vi "Auton - Boiler Shoot.vi"(10 "Alliance":T2, 11 "Auton States":T1=enum."Reset Encoders") -> ()   [LabVIEW 2016]
uses:
  Auton - Boiler Shoot States.ctl
  <vilib>/Rock Robotics/WPI/DriverStation/WPI_DriverStationAllianceInfo.ctl
  Robot Values.vi
panel:
  out "Auton State Current":T1=enum."Reset Encoders"
  in  "High Speed Output Range":cluster{"output high":dbl, "output low":dbl}={"output high"=0.9, "output low"=-0.9}
  in  "Cross Baseline SP":dbl=50.0
  in  "Turn to Zero SP (...)":dbl format="%#_13g"
  out "Original Time":timestamp
  in  "Back away  SP":dbl
  in  "Red - Turn Toward Angle SP":dbl=128.0
  in  "Approach Boiler SP":dbl=22.0
  in  "Blue - Turn Toward Angle SP":dbl=232.0
  in  "Initial Drive Forward SP":dbl=34.0
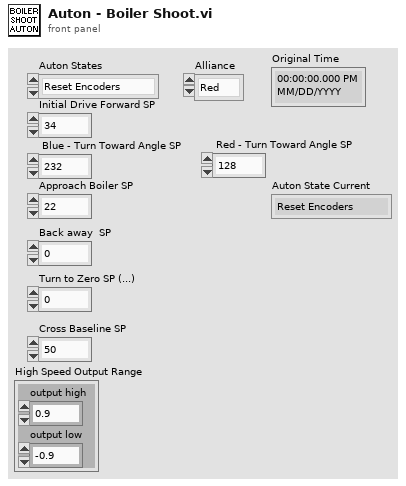
[diagram p1: front panel]
types:
  T1 = typedef "Auton - Boiler Shoot States.ctl" = enum16{"Stop", "Reset Encoders", "Drive Forward", "Turn toward boiler", "Reset Encoders Again", "Drive to boiler", "Shoot", "Back from Boiler", "Turn to Zero", "Reset Encoders Again Again", "Cross Baseline"}
  T2 = typedef "WPI_DriverStationAllianceInfo.ctl" = enum16{"Red", "Blue", "Invalid"}
  T3 = typedef "Robot Values.ctl" = cluster{"Robot Drive":cluster{"Left Motor Power":dbl, "Right Motor Power":dbl, "Left Encoder Value":dbl, "Right Encoder Value":dbl, "High Gear?":bool, "PTO?":bool}, "Sensors":cluster{"Gyro Angle":u16, "Recalibrate Gyro":bool, "Reset Gyro":bool, "Ultrasonic":dbl}, "Shooter":cluster{"Prep Wheels":bool, "Shoot":bool, "Left Shooter Wheel Speed":dbl, "Wheels Moving":bool, "Shooter Prepped":bool, "Shooter RPS SP":dbl, "Shooting?":bool, "Left Shooter Wheel Power":dbl, "Right Shooter Wheel Power":dbl, "Acquisition Conveyor Power":dbl, "Hopper Beater Bar Power":dbl, "Filtered Left Shooter Speed":dbl, "Acquisition Motor Power":dbl, "Joystick Add":dbl, "D-Pad Add":dbl, "Shooter Use PID?":bool}, "Robot States":cluster{"Drive mode":string, "Alliance":T2, "Position":T4}, "Gear":cluster{"Ejection Active":bool}}
  T4 = typedef "WPI_DriverStationPositionInfo.ctl" = enum16{"1", "2", "3"}
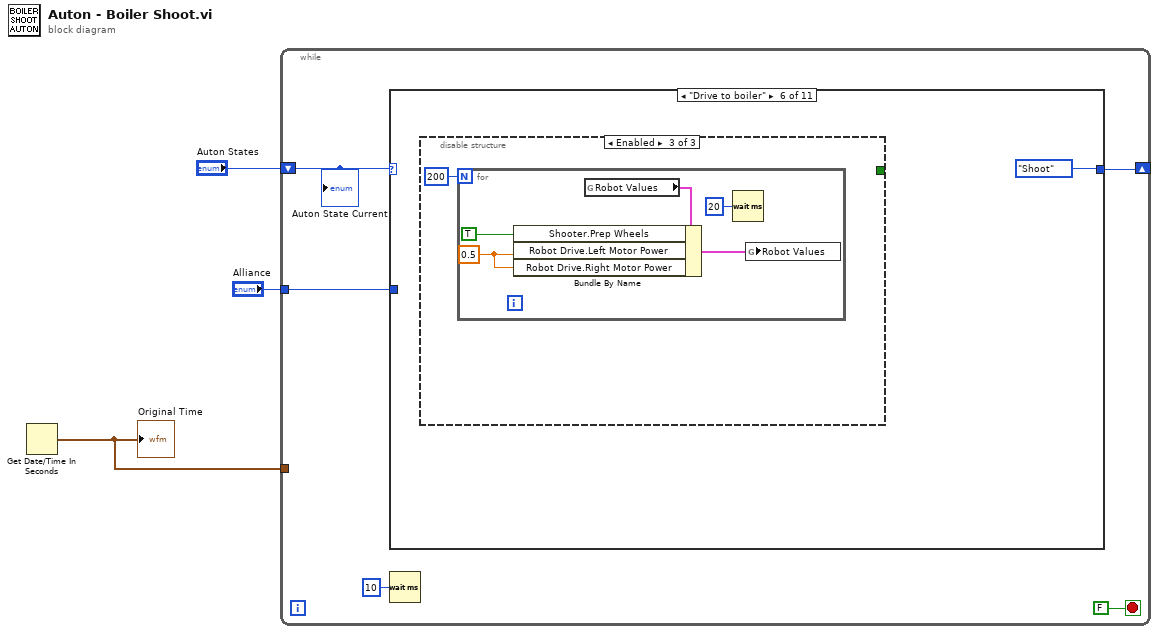
[diagram p0: block diagram]
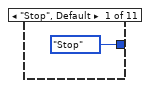
[diagram p2: hidden frame]
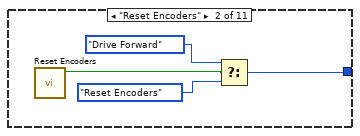
[diagram p3: hidden frame]
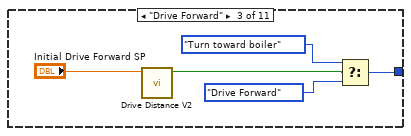
[diagram p4: hidden frame]
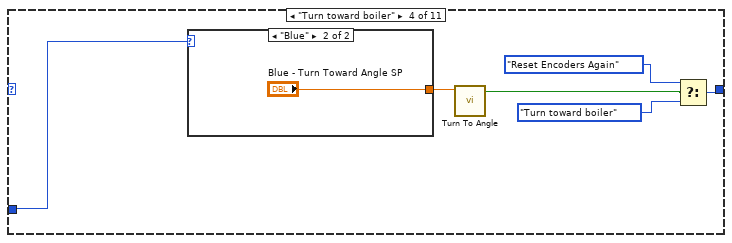
[diagram p5: hidden frame]
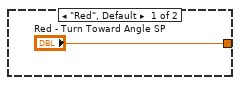
[diagram p6: hidden frame]
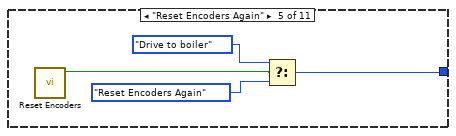
[diagram p7: hidden frame]
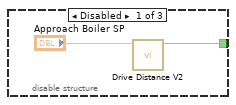
[diagram p8: hidden frame]
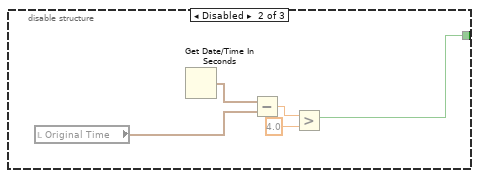
[diagram p9: hidden frame]
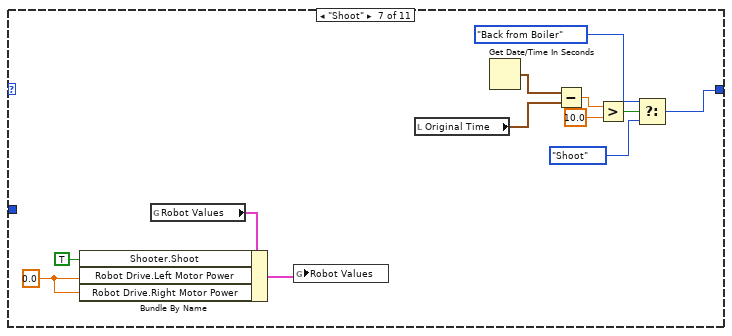
[diagram p10: hidden frame]
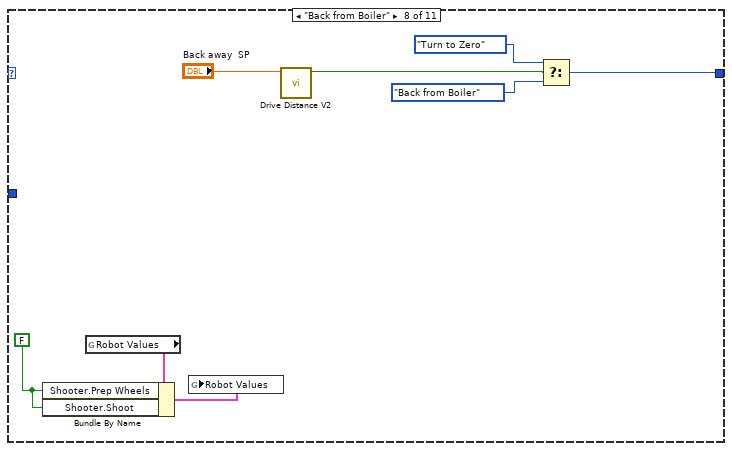
[diagram p11: hidden frame]
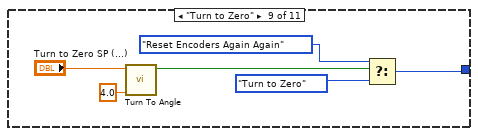
[diagram p12: hidden frame]
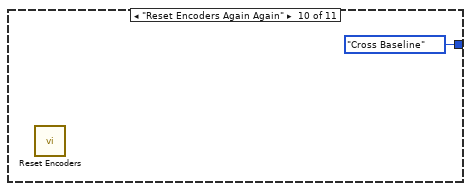
[diagram p13: hidden frame]
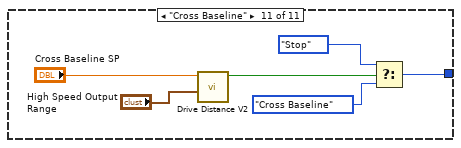
[diagram p14: hidden frame]
diagram:
  n1 = Get Date/Time In Seconds() -> (seconds since 1Jan1904=w1:timestamp)
  "Original Time" <- w1
  n2 = while {
    shift-right: [w7] -> _
    shift-left: "Auton States" -> [w8]
    tunnel: "Alliance" -> [w5]
    tunnel: w1 -> [_]
    stop <- FALSE stop-if-true
    n3 = case shown="\"Drive to boiler\"" w8 {
      tunnel: [Auton_-_Boiler_Shoot_States."Stop" ("Auton States") w10 w16 w22 w27 Auton_-_Boiler_Shoot_States."Shoot" ("Auton States") w48 w57 w69 Auton_-_Boiler_Shoot_States."Cross Baseline" ("f") w77] -> w7
      tunnel: w5 -> [_ _ _ w20 _ _ _ _ _ _ _]
      frame "Stop", Default {
      }
      frame "Reset Encoders" {
        n4 = call "Reset Encoders.vi"() -> ("Done?"=w13:bool)  [unwired: 11 in]
        n5 = Select(t=Auton_-_Boiler_Shoot_States."Drive Forward" ("Auton States"), s=w13, f=Auton_-_Boiler_Shoot_States."Reset Encoders" ("Auton States")) -> (s? t:f=w10:T1)
      }
      frame "Drive Forward" {
        n6 = call "Drive Distance V2.vi"("Distance Set Point"="Initial Drive Forward SP") -> ("Done?"=w15:bool)  [unwired: 10 in]
        n7 = Select(t=Auton_-_Boiler_Shoot_States."Turn toward boiler" ("Auton States"), s=w15, f=Auton_-_Boiler_Shoot_States."Drive Forward" ("Auton States")) -> (s? t:f=w16:T1)
      }
      frame "Turn toward boiler" {
        n8 = case shown="\"Blue\"" w20 {
          tunnel: ["Red - Turn Toward Angle SP" "Blue - Turn Toward Angle SP"] -> w19
          frame "Red", Default {
          }
          frame "Blue" {
          }
        }
        n9 = call "Turn To Angle.vi"("Setpoint"=w19) -> ("Done?"=w21:bool)  [unwired: 10 in]
        n10 = Select(t=Auton_-_Boiler_Shoot_States."Reset Encoders Again" ("Auton States"), s=w21, f=Auton_-_Boiler_Shoot_States."Turn toward boiler" ("Auton States")) -> (s? t:f=w22:T1)
      }
      frame "Reset Encoders Again" {
        n11 = call "Reset Encoders.vi"() -> ("Done?"=w30:bool)  [unwired: 11 in]
        n12 = Select(t=Auton_-_Boiler_Shoot_States."Drive to boiler" ("Auton States"), s=w30, f=Auton_-_Boiler_Shoot_States."Reset Encoders Again" ("Auton States")) -> (s? t:f=w27:T1)
      }
      frame "Drive to boiler" {
        n13 = disable-structure shown="Enabled" {
          disable-tunnel: [w33 w34 _] -> _
          frame Disabled {
            n14 = call "Drive Distance V2.vi"("Distance Set Point"="Approach Boiler SP") -> ("Done?"=w33:bool)  [unwired: 10 in]
          }
          frame Disabled {
            n15 = local read "Original Time"() -> (w35:timestamp)
            n16 = Get Date/Time In Seconds() -> (seconds since 1Jan1904=w38:timestamp)
            n17 = Subtract(x=w38, y=w35) -> (x-y=w37:dbl)
            n18 = Greater?(x=w37, y=4.0) -> (0:w34:bool)
          }
          frame Enabled {
            n19 = for {
              N: 200 -> [_]
              w43 = 0.5 ("Robot Drive.Left Motor Power")
              n20 = global read "Robot Values.vi" "Robot Values"() -> (w40:T3)
              n21 = Bundle By Name(cluster=w40, "Shooter.Prep Wheels"=TRUE, "Robot Drive.Left Motor Power"=w43, "Robot Drive.Right Motor Power"=w43) -> (w41:T3)
              n22 = Wait (ms)(milliseconds to wait=u32 20) -> ()  [unwired: 1 out]
              n23 = global write "Robot Values.vi" "Robot Values"(w41) -> ()
            }
          }
        }
      }
      frame "Shoot" {
        w45 = 0.0 ("Robot Drive.Left Motor Power")
        n24 = global read "Robot Values.vi" "Robot Values"() -> (w56:T3)
        n25 = Bundle By Name(cluster=w56, "Shooter.Shoot"=TRUE, "Robot Drive.Left Motor Power"=w45, "Robot Drive.Right Motor Power"=w45) -> (w55:T3)
        n26 = global write "Robot Values.vi" "Robot Values"(w55) -> ()
        n27 = local read "Original Time"() -> (w52:timestamp)
        n28 = Get Date/Time In Seconds() -> (seconds since 1Jan1904=w53:timestamp)
        n29 = Subtract(x=w53, y=w52) -> (x-y=w51:dbl)
        n30 = Greater?(x=w51, y=10.0) -> (0:w49:bool)
        n31 = Select(t=Auton_-_Boiler_Shoot_States."Back from Boiler", s=w49, f=Auton_-_Boiler_Shoot_States."Shoot" ("Auton States")) -> (s? t:f=w48:T1)
      }
      frame "Back from Boiler" {
        w62 = FALSE
        n32 = global read "Robot Values.vi" "Robot Values"() -> (w64:T3)
        n33 = Bundle By Name(cluster=w64, "Shooter.Prep Wheels"=w62, "Shooter.Shoot"=w62) -> (w63:T3)
        n34 = global write "Robot Values.vi" "Robot Values"(w63) -> ()
        n35 = call "Drive Distance V2.vi"("Distance Set Point"="Back away  SP") -> ("Done?"=w59:bool)  [unwired: 10 in]
        n36 = Select(t=Auton_-_Boiler_Shoot_States."Turn to Zero" ("Auton States"), s=w59, f=Auton_-_Boiler_Shoot_States."Back from Boiler" ("Auton States")) -> (s? t:f=w57:T1)
      }
      frame "Turn to Zero" {
        n37 = call "Turn To Angle.vi"("Turn Angle Tolerance"=4.0, "Setpoint"="Turn to Zero SP (...)") -> ("Done?"=w68:bool)  [unwired: 9 in]
        n38 = Select(t=Auton_-_Boiler_Shoot_States."Reset Encoders Again Again" ("Auton States"), s=w68, f=Auton_-_Boiler_Shoot_States."Turn to Zero") -> (s? t:f=w69:T1)
      }
      frame "Reset Encoders Again Again" {
        n39 = call "Reset Encoders.vi"() -> ()  [unwired: 11 in, 1 out]
      }
      frame "Cross Baseline" {
        n40 = call "Drive Distance V2.vi"("output range"="High Speed Output Range", "Distance Set Point"="Cross Baseline SP") -> ("Done?"=w75:bool)  [unwired: 9 in]
        n41 = Select(t=Auton_-_Boiler_Shoot_States."Stop" ("Auton States"), s=w75, f=Auton_-_Boiler_Shoot_States."Cross Baseline") -> (s? t:f=w77:T1)
      }
    }
    n42 = Wait (ms)(milliseconds to wait=u32 10) -> ()  [unwired: 1 out]
    "Auton State Current" <- w8
  }
